vi "PPSU Set parameters.vi"(7 "PPSU IP String":string, 8 "Error in":errorcluster, 10 "Data":T1, 11 "Device information array":string[][](array[string])) -> (0 "Fehler (Ausgang)":errorcluster caption="Error out", 3 "Device information out":string[](array[string]))   [LabVIEW 2022 SP3]
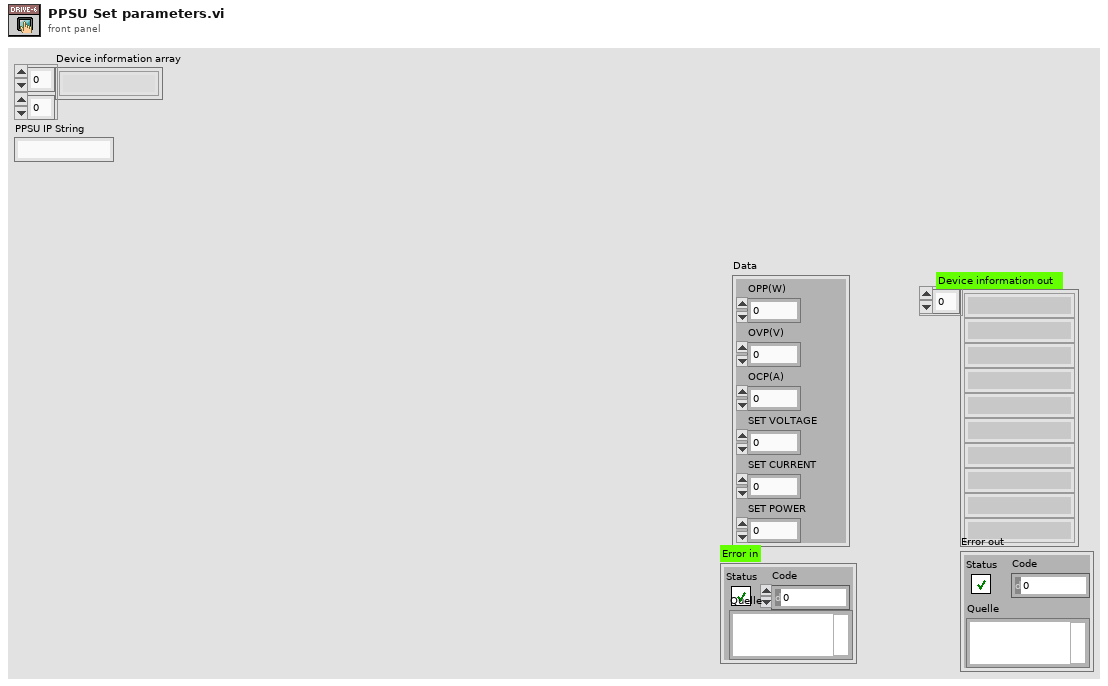
[diagram p1: front panel]
types:
  T1 = cluster{"OPP(W)":dbl, "OVP(V)":dbl, "OCP(A)":dbl, "SET VOLTAGE":dbl, "SET CURRENT":dbl, "SET POWER":dbl}
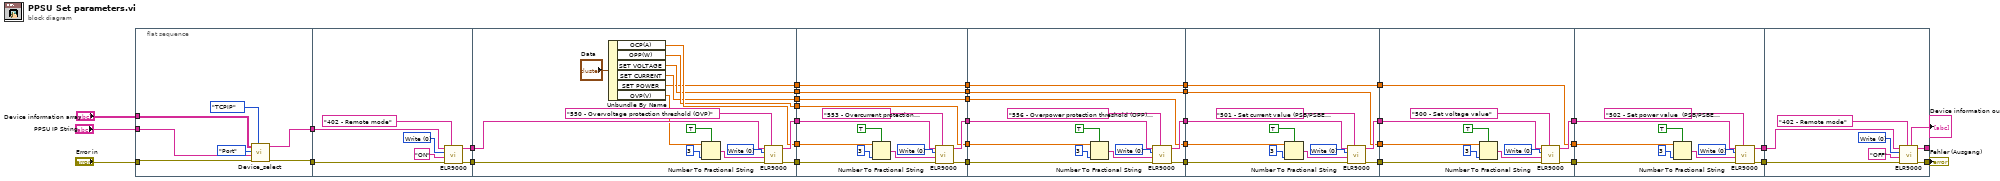
[diagram p0: block diagram]
diagram:
  n1 = flat-sequence {
    tunnel: "Error in" -> [w43]
    tunnel: [w42] -> w4
    tunnel: [w38] -> w3
    tunnel: "PPSU IP String" -> [w41]
    tunnel: "Device information array" -> [w39]
    tunnel: [w46] -> w36
    tunnel: [w45] -> w35
    tunnel: w4 -> [w50]
    tunnel: w3 -> [w44]
    tunnel: [w64] -> w34
    tunnel: [w63] -> w33
    tunnel: w36 -> [w62]
    tunnel: w35 -> [w61]
    tunnel: [w57] -> w32
    tunnel: [w56] -> w31
    tunnel: [w55] -> w30
    tunnel: [w54] -> w29
    tunnel: [w53] -> w28
    tunnel: w34 -> [w74]
    tunnel: w33 -> [w75]
    tunnel: [w73] -> w27
    tunnel: [w72] -> w26
    tunnel: w32 -> [w71]
    tunnel: [w70] -> w25
    tunnel: w31 -> [w70]
    tunnel: [w69] -> w24
    tunnel: w30 -> [w69]
    tunnel: [w68] -> w23
    tunnel: w29 -> [w68]
    tunnel: [w67] -> w22
    tunnel: w28 -> [w67]
    tunnel: w27 -> [w88]
    tunnel: w26 -> [w87]
    tunnel: [w86] -> w21
    tunnel: [w85] -> w20
    tunnel: w25 -> [w84]
    tunnel: [w83] -> w19
    tunnel: w24 -> [w83]
    tunnel: [w82] -> w18
    tunnel: w23 -> [w82]
    tunnel: [w81] -> w17
    tunnel: w22 -> [w81]
    tunnel: [w104] -> w16
    tunnel: [w103] -> w15
    tunnel: w21 -> [w98]
    tunnel: w20 -> [w97]
    tunnel: w19 -> [w96]
    tunnel: [w95] -> w14
    tunnel: w18 -> [w95]
    tunnel: [w94] -> w13
    tunnel: w17 -> [w94]
    tunnel: w16 -> [w109]
    tunnel: [w111] -> w12
    tunnel: w15 -> [w108]
    tunnel: [w110] -> w11
    tunnel: w14 -> [w107]
    tunnel: [w106] -> w10
    tunnel: w13 -> [w106]
    tunnel: w12 -> [w121]
    tunnel: [w119] -> w8
    tunnel: w11 -> [w120]
    tunnel: [w118] -> w9
    tunnel: w10 -> [w117]
    tunnel: w9 -> [w133]
    tunnel: w8 -> [w132]
    tunnel: [w128] -> w6
    tunnel: [w127] -> w5
    frame #0 {
      n2 = call <vilib>:"Device_select.vi"("Reference"=enum16{"ASRL/COM", "GPIB", "TCPIP"}."TCPIP", "error in (no error)"=w43, "Alias"=w41, "Open by"=enum16{"Device Node", "Serial number", "Port"}."Port", "Device information array"=w39) -> ("error out"=w42:errorcluster, "Device information"=w38:string[])  [unwired: 2 in]
    }
    frame #1 {
      w48 = u8 0 items=["Write", "Read"] ("Access")
      n3 = call <vilib>:"ELR9000.vi"("Command list"="402 - Remote mode", "Error in"=w50, "Value"="ON", "Access"=w48, "Device information in"=w44) -> ("Error out"=w45:errorcluster, "Device information out"=w46:string[])  [unwired: 1 in, 2 out]
    }
    frame #2 {
      w66 = u8 0 items=["Write", "Read"] ("Access")
      n4 = Unbundle By Name("Data") -> ("OCP(A)"=w57:dbl, "OPP(W)"=w56:dbl, "SET VOLTAGE"=w54:dbl, "SET CURRENT"=w55:dbl, "SET POWER"=w53:dbl, "OVP(V)"=w52:dbl)
      n5 = Number To Fractional String(use system decimal point (T)=TRUE, number=w52, precision (6)=i16 3) -> (F-format string=w58:string)  [unwired: 1 in]
      n6 = call <vilib>:"ELR9000.vi"("Command list"="550 - Overvoltage protection threshold (OVP)", "Error in"=w61, "Value"=w58, "Access"=w66, "Device information in"=w62) -> ("Error out"=w64:errorcluster, "Device information out"=w63:string[])  [unwired: 1 in, 2 out]
    }
    frame #3 {
      w80 = u8 0 items=["Write", "Read"] ("Access")
      n7 = Number To Fractional String(use system decimal point (T)=TRUE, number=w71, precision (6)=i16 3) -> (F-format string=w76:string)  [unwired: 1 in]
      n8 = call <vilib>:"ELR9000.vi"("Command list"="553 - Overcurrent protection threshold (OCP) (PSB/PSBE devices: source mode)", "Error in"=w74, "Value"=w76, "Access"=w80, "Device information in"=w75) -> ("Error out"=w72:errorcluster, "Device information out"=w73:string[])  [unwired: 1 in, 2 out]
    }
    frame #4 {
      w93 = u8 0 items=["Write", "Read"] ("Access")
      n9 = Number To Fractional String(use system decimal point (T)=TRUE, number=w84, precision (6)=i16 3) -> (F-format string=w89:string)  [unwired: 1 in]
      n10 = call <vilib>:"ELR9000.vi"("Command list"="556 - Overpower protection threshold (OPP) (PSB/PSBE devices: source mode)", "Error in"=w87, "Value"=w89, "Access"=w93, "Device information in"=w88) -> ("Error out"=w85:errorcluster, "Device information out"=w86:string[])  [unwired: 1 in, 2 out]
    }
    frame #5 {
      w105 = u8 0 items=["Write", "Read"] ("Access")
      n11 = Number To Fractional String(use system decimal point (T)=TRUE, number=w96, precision (6)=i16 3) -> (F-format string=w99:string)  [unwired: 1 in]
      n12 = call <vilib>:"ELR9000.vi"("Command list"="501 - Set current value (PSB/PSBE devices: source mode) / Irradiation (PV function, PSI/PSB only) ", "Error in"=w97, "Value"=w99, "Access"=w105, "Device information in"=w98) -> ("Error out"=w103:errorcluster, "Device information out"=w104:string[])  [unwired: 1 in, 2 out]
    }
    frame #6 {
      w116 = u8 0 items=["Write", "Read"] ("Access")
      n13 = Number To Fractional String(use system decimal point (T)=TRUE, number=w107, precision (6)=i16 3) -> (F-format string=w112:string)  [unwired: 1 in]
      n14 = call <vilib>:"ELR9000.vi"("Command list"="500 - Set voltage value", "Error in"=w108, "Value"=w112, "Access"=w116, "Device information in"=w109) -> ("Error out"=w110:errorcluster, "Device information out"=w111:string[])  [unwired: 1 in, 2 out]
    }
    frame #7 {
      w126 = u8 0 items=["Write", "Read"] ("Access")
      n15 = Number To Fractional String(use system decimal point (T)=TRUE, number=w117, precision (6)=i16 3) -> (F-format string=w122:string)  [unwired: 1 in]
      n16 = call <vilib>:"ELR9000.vi"("Command list"="502 - Set power value  (PSB/PSBE devices: source mode)", "Error in"=w120, "Value"=w122, "Access"=w126, "Device information in"=w121) -> ("Error out"=w118:errorcluster, "Device information out"=w119:string[])  [unwired: 1 in, 2 out]
    }
    frame #8 {
      w130 = u8 0 items=["Write", "Read"] ("Access")
      n17 = call <vilib>:"ELR9000.vi"("Command list"="402 - Remote mode", "Error in"=w133, "Value"="OFF", "Access"=w130, "Device information in"=w132) -> ("Error out"=w127:errorcluster, "Device information out"=w128:string[])  [unwired: 1 in, 2 out]
    }
  }
  "Device information out" <- w6
  "Fehler (Ausgang)" <- w5
